vi "stop test after prompt.vi"(8 "error in":errorcluster, 10 "step_description (prompt)":string, 11 "test control queue":refnum<queue>) -> (0 "error out":errorcluster, 3 "test control queue out":refnum<queue>)   [LabVIEW 2020]
uses:
  controls/test control.ctl
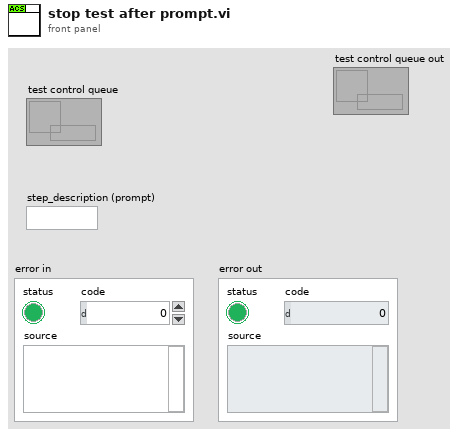
[diagram p1: front panel]
types:
  T1 = typedef "test control.ctl" = cluster{"Exit Program":bool, "Stop Test":bool, "Start Test":bool}
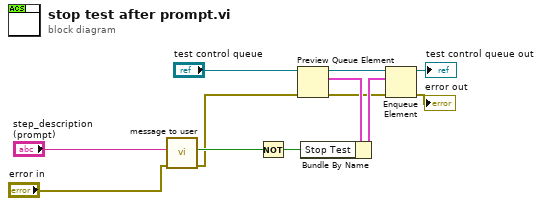
[diagram p0: block diagram]
diagram:
  n1 = call "message to user.vi"("error in (no error)"="error in", "step_description (prompt)"="step_description (prompt)") -> ("error out"=w3:errorcluster, "OK"=w11:bool)  [unwired: 8 in]
  n2 = Not(x=w11) -> (.not. x?=w12:bool)
  n3 = Preview Queue Element(queue="test control queue", error in (no error)=w3) -> (queue out=w7:refnum<queue>, element=w6:T1, error out=w2:errorcluster)  [unwired: 1 in, 1 out]
  n4 = Bundle By Name(cluster=w6, "Stop Test"=w12) -> (w10:T1)
  n5 = Enqueue Element(queue=w7, element=w10, error in (no error)=w2) -> (queue out=→"test control queue out":refnum<queue>, error out=→"error out":errorcluster)  [unwired: 1 in, 1 out]
